vi "Segmented Array Average.vi"(9 "Sub Sampling Interval":i32, 11 "Data":dbl[](array[numeric])) -> (3 "Segmented Average":dbl)   [LabVIEW 2018]
uses:
  ffcfc141-4f8f-4e33-ae38-9b58b20249bc.vi
  dddf362e-cda5-4bfd-adc4-65125c071599.vi
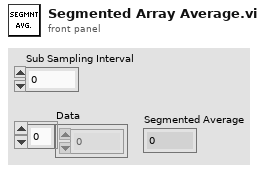
[diagram p1: front panel]
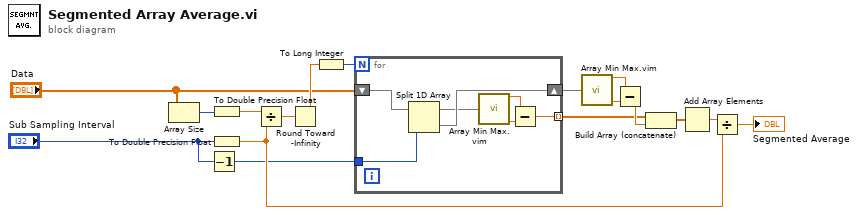
[diagram p0: block diagram]
diagram:
  n1 = Array Size(array="Data") -> (size(s)=w3:i32)
  n2 = Decrement(x="Sub Sampling Interval") -> (x-1=w8:i32)
  n3 = To Double Precision Float(number=w3) -> (double precision float=w6:dbl)
  n4 = To Double Precision Float(number="Sub Sampling Interval") -> (double precision float=w16:dbl)
  n5 = Divide(x=w6, y=w16) -> (x/y=w4:dbl)
  n6 = Round Toward -Infinity(1:w4) -> (0:w5:dbl)
  n7 = To Long Integer(number=w5) -> (32bit integer=w7:i32)
  n8 = for {
    N: w7 -> [_]
    shift-right: [w23] -> w9
    shift-left: "Data" -> [w24]
    tunnel: w8 -> [w22]
    tunnel: [w18] -> w12 mode=indexing
    n9 = Split 1D Array(array=w24, index=w22) -> (first subarray=w21:dbl[], second subarray=w23:dbl[])
    n10 = call "Array Min Max.vim"("Array"=w21) -> ("Max"=w20:dbl, "Min"=w19:dbl)  [unwired: 13 in]
    n11 = Subtract(x=w20, y=w19) -> (x-y=w18:dbl)
  }
  n12 = call "Array Min Max.vim"("Array"=w9) -> ("Max"=w10:dbl, "Min"=w11:dbl)  [unwired: 13 in]
  n13 = Subtract(x=w10, y=w11) -> (x-y=w13:dbl)
  n14 = Build Array (concatenate)(w12, w13) -> (w14:dbl[])
  n15 = Add Array Elements(numeric array=w14) -> (sum=w17:dbl)
  n16 = Divide(x=w17, y=w16) -> (x/y=→"Segmented Average":dbl)
